vi "CAMERA_task_DONE.vi"(1 "error in":errorcluster) -> (0 "error out":errorcluster)   [LabVIEW 2015]
uses:
  <vilib>/Utility/error.llb/DialogType.ctl
  GLOBAL/Global_CAMERA.vi
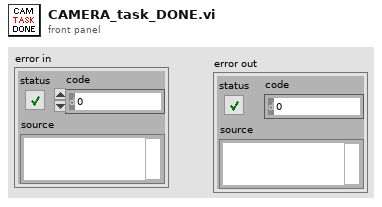
[diagram p1: front panel]
types:
  T1 = typedef "DialogType.ctl" = u16
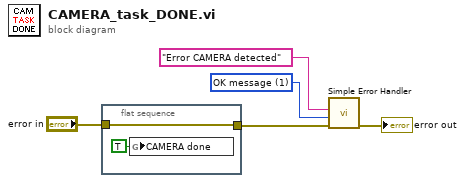
[diagram p0: block diagram]
diagram:
  w2 = T1 1 items=["no dialog", "OK message", "continue or stop message", "OK message + warnings", "continue/stop + warnings"] ("type of dialog (OK msg:1)")
  n1 = flat-sequence {
    tunnel: "error in" -> [w6]
    tunnel: [w6] -> w4
    frame #0 {
      n2 = global write "Global_CAMERA.vi" "CAMERA done"(TRUE ("Start ANDOR")) -> ()
    }
  }
  n3 = call <vilib>:"Simple Error Handler.vi"("error source (\" \")"="Error CAMERA detected" ("error source (\" \")"), "type of dialog (OK msg:1)"=w2, "error in (no error)"=w4) -> ("error out"=→"error out":errorcluster)  [unwired: 2 in, 4 out]
